vi "read_master_file.vi"(8 "error in (no error)":errorcluster, 11 "master file path":string) -> (0 "error out":errorcluster, 3 "setup file paths":string)   [LabVIEW 2017, in "worker.lvlib"]
uses:
  worker.lvlib
  support/my_global.vi
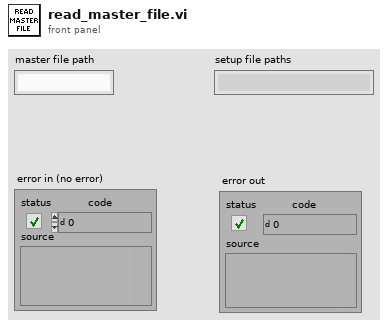
[diagram p1: front panel]
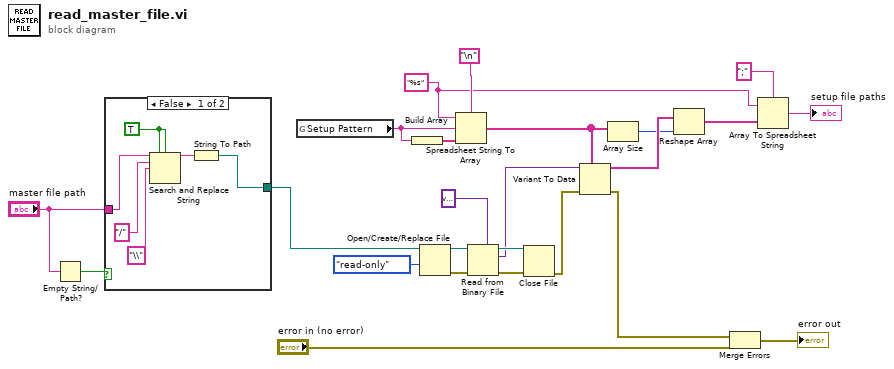
[diagram p0: block diagram]
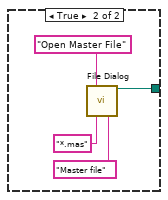
[diagram p2: hidden frame]
diagram:
  w10 = "%s" ("format string")
  n1 = Empty String/Path?(string/path="master file path") -> (empty?=w4:bool)
  n2 = case shown="False" w4 {
    tunnel: [w30 w33] -> w3
    tunnel: "master file path" -> [w29 _]
    frame False {
      w26 = TRUE ("replace all? (F)")
      n3 = Search and Replace String(replace all?=w26, case sensitive?=w26, input string=w29, search string="/", replace string="\\" ("replace string (\"\")")) -> (result string=w25:string)  [unwired: 3 in, 3 out]
      n4 = String To Path(string=w25) -> (path=w30:path)
    }
    frame True {
      n5 = call "File Dialog"("prompt"="Open Master File", "pattern (all files)"="*.mas", "pattern label"="Master file") -> ("selected path"=w33:path)  [unwired: 9 in, 3 out]
    }
  }
  n6 = global read "my_global.vi" "Setup Pattern"() -> (w17:string)
  n7 = Build Array(w17) -> (w16:string[])
  n8 = Open/Create/Replace File(file path (use dialog)=w3, access (0:read/write)=enum16{"read/write", "read-only", "write-only"}."read-only") -> (refnum out=w22:refnum<file>, error out=w23:errorcluster)  [unwired: 4 in, 1 out]
  n9 = Spreadsheet String To Array(delimiter (Tab)="\n", format string=w10, spreadsheet string=w17, array type (2D Dbl)=w16) -> (array=w14:string[])
  n10 = Read from Binary File(5:variant, 8:w23, 11:w22) -> (0:w20:errorcluster, 2:w18:variant, 3:w19:refnum<file>)  [unwired: 3 in, 1 out]
  n11 = Close File(refnum=w19, error in=w20) -> (error out=w8:errorcluster)  [unwired: 1 out]
  n12 = Variant To Data(error in=w8, type=w14, Variant=w18) -> (data=w15:string[], error out=w5:errorcluster)
  n13 = Array Size(array=w14) -> (size(s)=w13:i32)
  n14 = Reshape Array(w15, w13) -> (w12:string[])
  n15 = Merge Errors(w5, "error in (no error)") -> (→"error out":errorcluster)
  n16 = Array To Spreadsheet String(delimiter (Tab)=";", array=w12, 3:w10) -> (spreadsheet string=→"setup file paths":string)
